vi "ReadTreeStrict.vi"(8 "error in (no error)":errorcluster, 11 "ClassDataTree in":refnum<class "ClassDataTree.lvclass">) -> (0 "error out":errorcluster, 2 "Tree":refnum<vi>, 3 "ClassDataTree out":refnum<class "ClassDataTree.lvclass">)   [LabVIEW 2010, in "ClassDataTree.lvclass"]
uses:
  ClassDataTree.lvclass
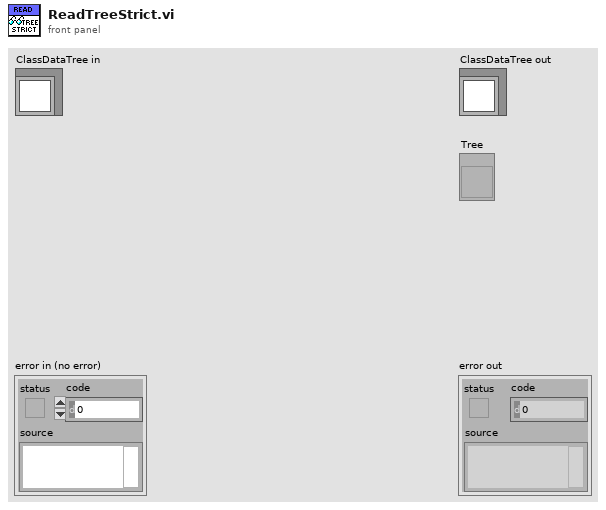
[diagram p1: front panel]
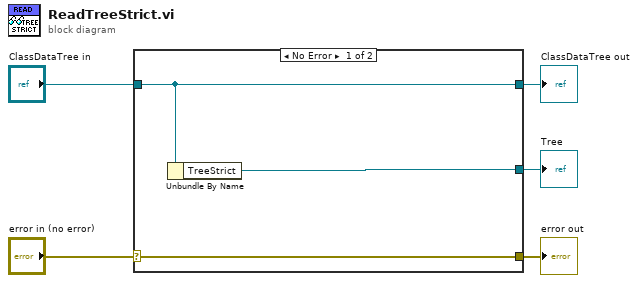
[diagram p0: block diagram]
diagram:
  n1 = case shown="No Error" "error in (no error)" {
    selector: "error in (no error)" -> [w8 w9]
    tunnel: [w8 w9] -> w4
    tunnel: [w7 w10] -> w2
    tunnel: "ClassDataTree in" -> [w7 w10]
    tunnel: [w6 _] -> w1
    frame No Error {
      n2 = Unbundle By Name(w7) -> ("TreeStrict"=w6:refnum<vi>)
    }
    frame Error {
    }
  }
  "error out" <- w4
  "ClassDataTree out" <- w2
  "Tree" <- w1
